vi "Execute.vi"(8 "error in":errorcluster, 9 "Consumer Queues in":T1, 10 "DAC Process Command in":refnum<class "Save DAC Configuration.lvclass">, 11 "DAC Process Data in":T2) -> (0 "error out":errorcluster, 1 "Consumer Queues out":T1, 2 "Stop?":bool, 3 "DAC Process Data out":T2)   [LabVIEW 2019, in "DAC Process.lvlib" / "Save DAC Configuration.lvclass"]
uses:
  Save DAC Configuration.lvclass
  DAC Process Data.ctl
  Generic Test Stand/Generic Test Stand.lvclass
  TS Framework/ExeLogging/DAC Logger/DAC Logger.lvclass
  DAC State.ctl
  TS Framework/Consumer Queues.ctl
  UI Process/Generic UI Command/Generic UI Process Command.lvclass
  Generic DAC Command/Generic DAC Process Command.lvclass
  Trig Process/Generic Trig Command/Generic Trig Process Command.lvclass
  DAC Process.lvlib
  TS Framework/TS Framework.lvlib
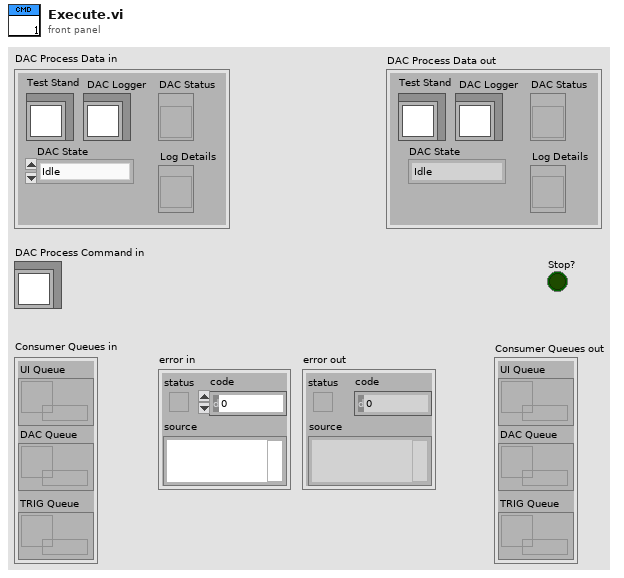
[diagram p1: front panel]
types:
  T1 = typedef "TS Framework.lvlib/Consumer Queues.ctl" = cluster{"UI Queue":refnum<queue>, "DAC Queue":refnum<queue>, "TRIG Queue":refnum<queue>}
  T2 = typedef "DAC Process.lvlib/DAC Process Data.ctl" = cluster{"Test Stand":refnum<class "Generic Test Stand.lvclass">, " DAC Logger":refnum<class "DAC Logger.lvclass">, "DAC State":T3, "DAC Status":refnum<vi>, "Log Details":refnum<vi>}
  T3 = typedef "DAC Process.lvlib/DAC State.ctl" = enum16{"Idle", "Acquiring"}
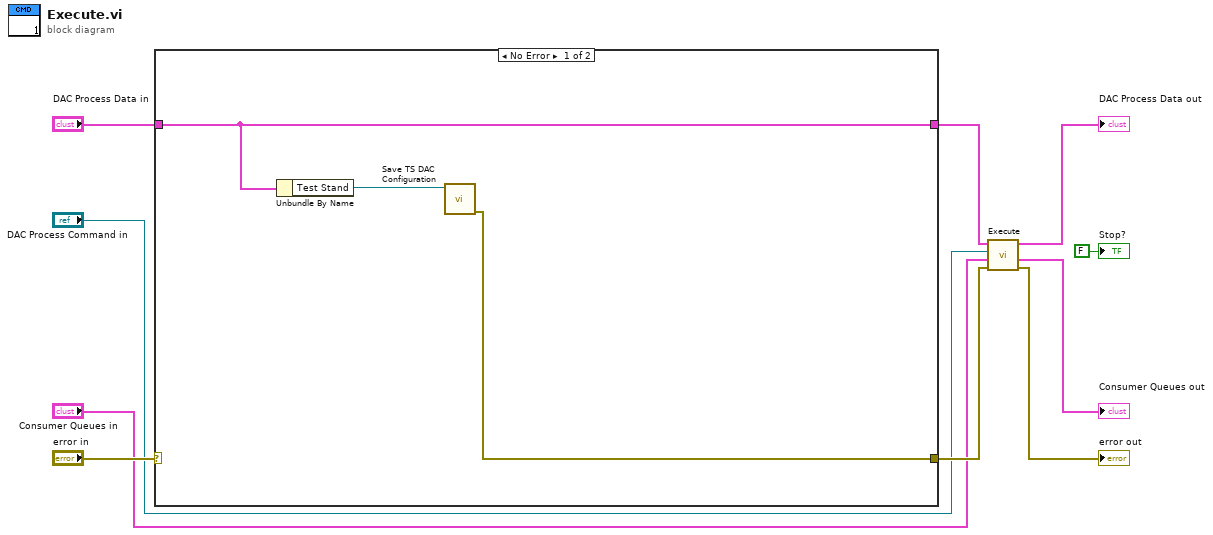
[diagram p0: block diagram]
diagram:
  n1 = case shown="No Error" "error in" {
    selector: "error in" -> [_ w15]
    tunnel: [w11 w15] -> w5
    tunnel: "DAC Process Data in" -> [w13 w14]
    tunnel: [w13 w14] -> w3
    frame No Error {
      n2 = Unbundle By Name(w13) -> ("Test Stand"=w12:refnum<class "Generic Test Stand.lvclass">)
      n3 = call-dynamic "Save TS DAC Configuration.vi"("Generic Test Stand in"=w12) -> ("error out"=w11:errorcluster)  [unwired: 9 in, 1 out]
    }
    frame Error {
    }
  }
  n4 = call-parent "Execute.vi"("error in"=w5, "Consumer Queues in"="Consumer Queues in", "DAC Process Command in"="DAC Process Command in", "DAC Process Data in"=w3) -> ("error out"=→"error out":errorcluster, "Consumer Queues out"=→"Consumer Queues out":T1, "DAC Process Data out"=→"DAC Process Data out":T2)  [unwired: 4 in, 1 out]
  "Stop?" <- FALSE ("Stop?")
